vi "Collect Numeric Array(DBL).vi"(6 "reset":bool, 7 "enable":bool=TRUE, 8 "error in":errorcluster, 10 "array size":u32=10, 11 "input":dbl) -> (0 "error out":errorcluster, 1 "full":bool, 2 "points collected":i32=10, 3 "collected data":dbl[](array[numeric]))   [LabVIEW 2012]
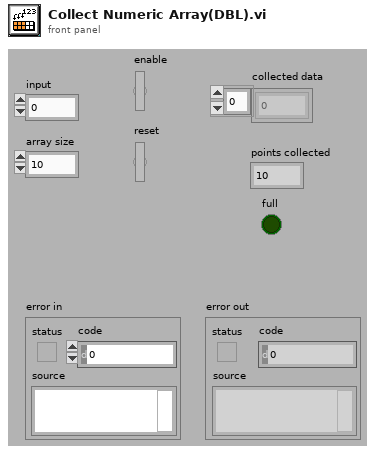
[diagram p1: front panel]
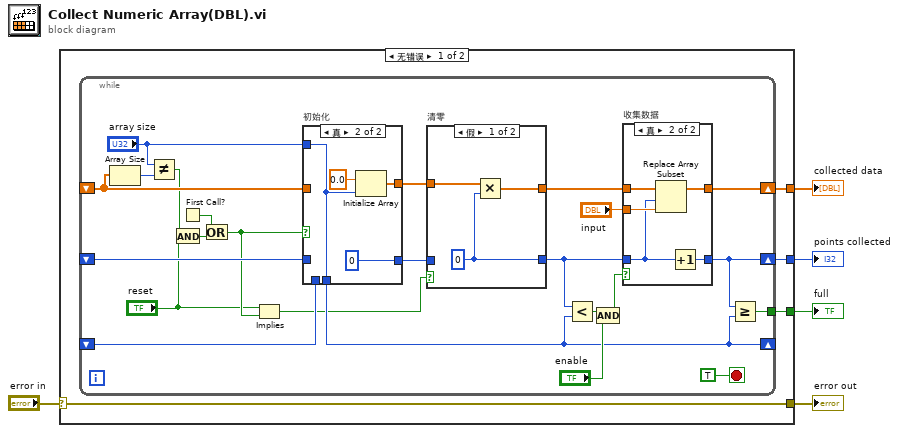
[diagram p0: block diagram]
diagram:
  n1 = case shown="无错误" "error in" {
    selector: "error in" -> [w7 w53]
    tunnel: [w9 _] -> w5
    tunnel: [w6 _] -> w4
    tunnel: [w8 _] -> w3
    tunnel: [w7 w53] -> w1
    frame No Error {
      n2 = while {
        shift-right: [w33] -> w9
        shift-left: _ -> [w19]
        shift-right: [w22] -> w8
        shift-left: _ -> [w31]
        shift-right: [w21] -> _
        shift-left: _ -> [w32]
        tunnel: [w10] -> w6
        stop <- TRUE stop-if-true
        n3 = Array Size(array=w19) -> (size(s)=w18:i32)
        n4 = Not Equal?(x="array size", y=w18) -> (x != y?=w16:bool)
        n5 = And(x=w16, y="reset") -> (x .and. y?=w15:bool)
        n6 = First Call?() -> (First Call?: T/F=w14:bool)
        n7 = Or(x=w14, y=w15) -> (x .or. y?=w13:bool)
        n8 = Implies(1:w13, 2:"reset") -> (0:w11:bool)
        n9 = case "初始化" shown="真" w13 {
          tunnel: "array size" -> [_ w49]
          tunnel: [w46 0] -> w28
          tunnel: [w47 w50] -> w26
          tunnel: [w48 w49] -> w21
          tunnel: w32 -> [w48 _]
          tunnel: w19 -> [w47 _]
          tunnel: w31 -> [w46 _]
          frame False {
          }
          frame True {
            n10 = Initialize Array(0.0 ("element"), w49) -> (w50:dbl[])
          }
        }
        n11 = case "清零" shown="假" w11 {
          tunnel: w28 -> [_ w38]
          tunnel: [w34 w38] -> w27
          tunnel: w26 -> [w36 w37]
          tunnel: [w35 w37] -> w25
          frame False {
            w34 = 0
            n12 = Multiply(x=w36, y=w34) -> (x*y=w35:dbl[])
          }
          frame True {
          }
        }
        n13 = Less?(x=w27, y=w21) -> (x < y?=w20:bool)
        n14 = Compound Arithmetic op=AND(w20, "enable") -> (w30:bool)
        n15 = case "收集数据" shown="真" w30 {
          tunnel: "input" -> [_ w45]
          tunnel: w27 -> [w39 w42]
          tunnel: w25 -> [w40 w44]
          tunnel: [w40 w43] -> w33
          tunnel: [w39 w41] -> w22
          frame False {
          }
          frame True {
            n16 = Replace Array Subset(array=w44, new element=w45, index=w42) -> (w43:dbl[])
            n17 = Increment(x=w42) -> (x+1=w41:i32)
          }
        }
        n18 = Greater Or Equal?(x=w22, y=w21) -> (x >= y?=w10:bool)
      }
    }
    frame Error {
    }
  }
  "collected data" <- w5
  "full" <- w4
  "points collected" <- w3
  "error out" <- w1
